vi "config.vi"(8 "error in (no error)":errorcluster, 11 "Keithley2002 in":refnum<class "Keithley2002.lvclass">) -> (0 "error out":errorcluster, 3 "Keithley2002 out":refnum<class "Keithley2002.lvclass">)   [LabVIEW 2019, in "Keithley2002.lvclass"]
uses:
  Keithley2002.lvclass
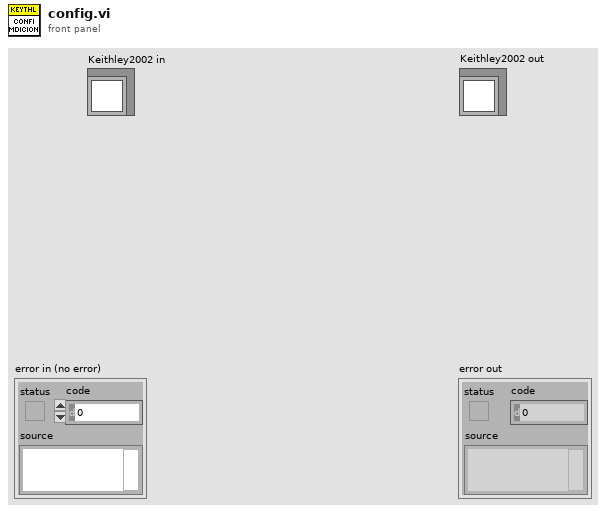
[diagram p1: front panel]
types:
  T1 = cluster{"error":bool, "code":i32, "source":string}
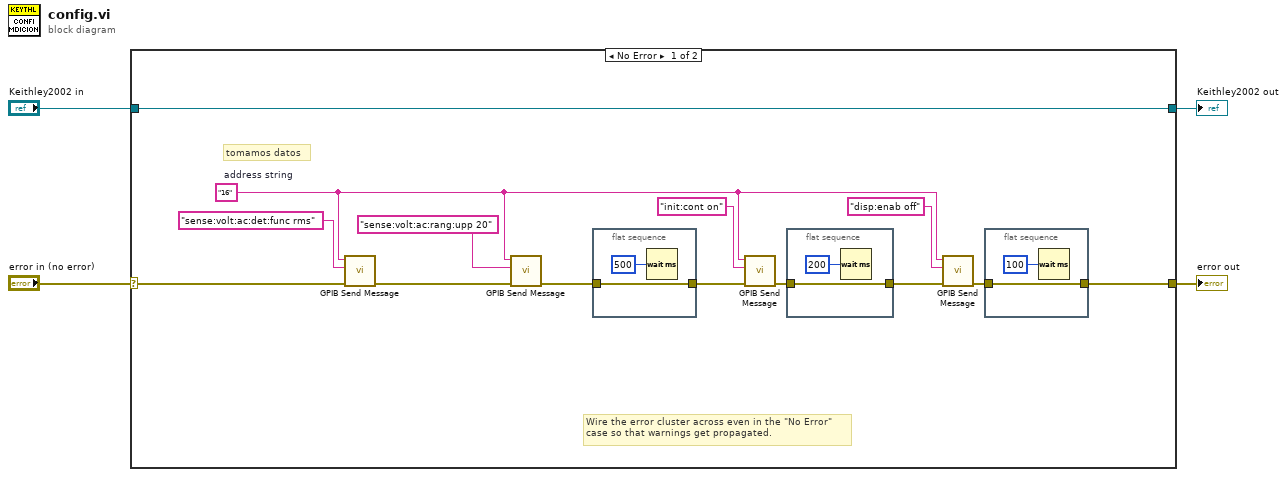
[diagram p0: block diagram]
diagram:
  n1 = case shown="No Error" "error in (no error)" {
    selector: "error in (no error)" -> [w6 w26]
    tunnel: [w5 w26] -> w3
    tunnel: [w18 w25] -> w1
    tunnel: "Keithley2002 in" -> [w18 w25]
    frame No Error {
      w7 = "16"  # address string
      # "tomamos datos"
      # "Wire the error cluster across even in the \"No Error\"\ncase so that warnings get propagated."
      n2 = call <instrlib>:"GPIB Send Message.vi"("address string"=w7, "write buffer"="sense:volt:ac:det:func rms", "error in"=w6) -> ("error out"=w14:T1)  [unwired: 4 in, 2 out]
      n3 = call <instrlib>:"GPIB Send Message.vi"("address string"=w7, "write buffer"="sense:volt:ac:rang:upp 20", "error in"=w14) -> ("error out"=w9:T1)  [unwired: 4 in, 2 out]
      n4 = flat-sequence {
        tunnel: w9 -> [w24]
        tunnel: [w24] -> w13
        frame #0 {
          n5 = Wait (ms)(milliseconds to wait=u32 500) -> ()  [unwired: 1 out]
        }
      }
      n6 = call <instrlib>:"GPIB Send Message.vi"("address string"=w7, "write buffer"="init:cont on", "error in"=w13) -> ("error out"=w12:T1)  [unwired: 4 in, 2 out]
      n7 = flat-sequence {
        tunnel: w12 -> [w22]
        tunnel: [w22] -> w11
        frame #0 {
          n8 = Wait (ms)(milliseconds to wait=u32 200) -> ()  [unwired: 1 out]
        }
      }
      n9 = call <instrlib>:"GPIB Send Message.vi"("address string"=w7, "write buffer"="disp:enab off", "error in"=w11) -> ("error out"=w10:T1)  [unwired: 4 in, 2 out]
      n10 = flat-sequence {
        tunnel: w10 -> [w20]
        tunnel: [w20] -> w5
        frame #0 {
          n11 = Wait (ms)(milliseconds to wait=u32 100) -> ()  [unwired: 1 out]
        }
      }
    }
    frame Error {
    }
  }
  "error out" <- w3
  "Keithley2002 out" <- w1
